vi "PickGitInstall.vi"(8 "error in (no error)":errorcluster, 11 "Git Installs":path[](array[path])) -> (0 "error out":errorcluster, 2 "User Cancelled":bool, 3 "Git Path":path)   [LabVIEW 2013]
panel:
  in  "Cancel Button":bool
  in  "OK Button":bool
  in  "Choose your git installation":i32(listbox)
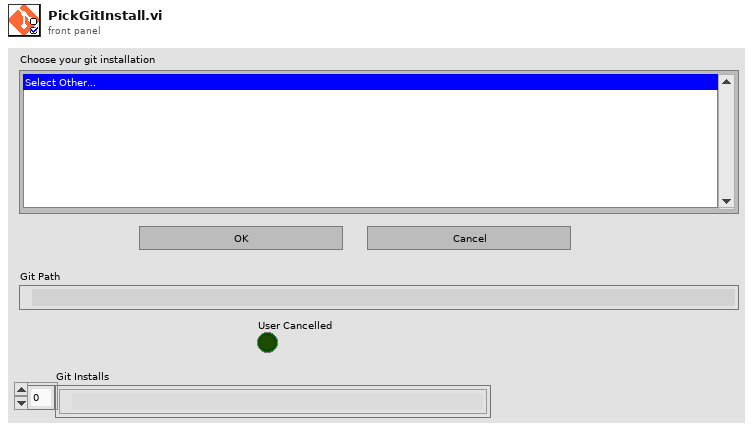
[diagram p1: front panel]
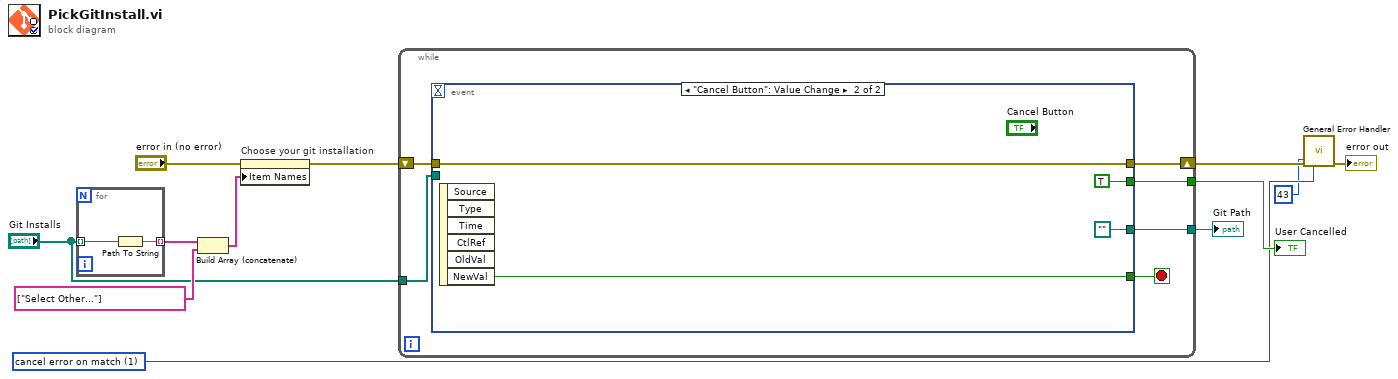
[diagram p0: block diagram]
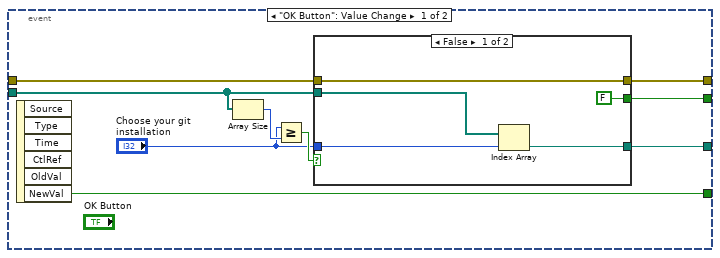
[diagram p2: hidden frame]
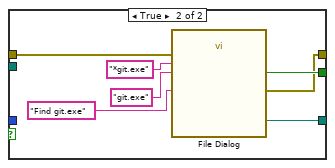
[diagram p3: hidden frame]
diagram:
  w2 = 1 items=["no exception", "cancel error on match", "set error on match"] ("[exception action] (none:0)")
  n1 = for {
    tunnel: "Git Installs" -> [w14] mode=indexing
    tunnel: [w13] -> w9 mode=indexing
    n2 = Path To String(path=w14) -> (string=w13:string)
  }
  n3 = Build Array (concatenate)(w9, string[] ["Select Other..."] ("element")) -> (w10:string[])
  n4 = property on="Choose your git installation" class="LstBox (strict)"(error in="error in (no error)", "Item Names"=w10) -> (error out=w8:errorcluster)  [unwired: 1 in, 1 out]
  n5 = while {
    shift-right: [w16] -> w4
    shift-left: w8 -> [w15]
    tunnel: [w19] -> w7
    tunnel: "Git Installs" -> [w18]
    tunnel: [w17] -> w5
    stop <- w20 stop-if-true
    n6 = event shown="[1] \"Cancel Button\": Value Change" {
      selector: _ -> [_ _]
      dyn-events: _ -> [_ _]
      timeout: _ -> [_ _]
      tunnel: [w29 w45] -> w20
      tunnel: [w24 path ""] -> w19
      tunnel: w18 -> [w26 _]
      tunnel: [w23 TRUE ("cancelled")] -> w17
      tunnel: [w22 w44] -> w16
      tunnel: w15 -> [w21 w44]
      event "OK Button": Value Change {
        n7 = event-data() -> ("NewVal"=w29:bool)  [unwired: 1 in, 5 out]
        n8 = Array Size(array=w26) -> (size(s)=w28:i32)
        n9 = Greater Or Equal?(x="Choose your git installation", y=w28) -> (x >= y?=w27:bool)
        n10 = case shown="False" w27 {
          tunnel: w26 -> [w34 _]
          tunnel: "Choose your git installation" -> [w33 _]
          tunnel: [w32 w38] -> w24
          tunnel: [FALSE w39] -> w23
          tunnel: [w30 w36] -> w22
          tunnel: w21 -> [w30 w35]
          frame False {
            n11 = Index Array(array=w34, index=w33) -> (element=w32:path)
          }
          frame True {
            n12 = call "File Dialog"("prompt"="Find git.exe", "error in"=w35, "pattern (all files)"="*git.exe", "pattern label"="git.exe") -> ("selected path"=w38:path, "cancelled"=w39:bool, "error out"=w36:errorcluster)  [unwired: 8 in, 1 out]
          }
        }
      }
      event "Cancel Button": Value Change {
        n13 = event-data() -> ("NewVal"=w45:bool)  [unwired: 1 in, 5 out]
      }
    }
  }
  "Git Path" <- w7
  "User Cancelled" <- w5
  n14 = call <vilib>:"General Error Handler.vi"("error in (no error)"=w4, "[exception action] (none:0)"=w2, "[exception code]"=43) -> ("error out"=→"error out":errorcluster)  [unwired: 8 in, 4 out]
